vi "Show Block Diagram.vi"(8 "error in":errorcluster, 11 "VI in":refnum<vi>) -> (0 "error out":errorcluster)   [LabVIEW 2014, in "Chart Module.lvlib"]
uses:
  Chart Module.lvlib
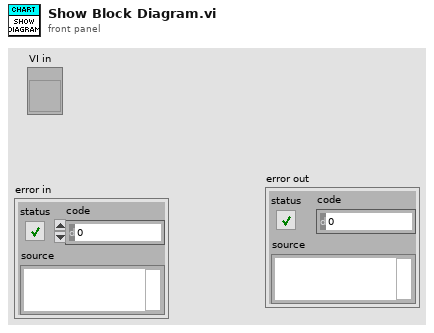
[diagram p1: front panel]
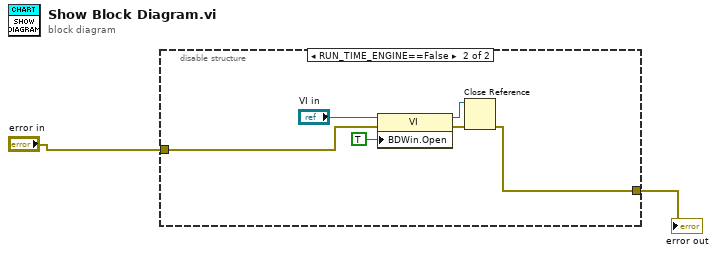
[diagram p0: block diagram]
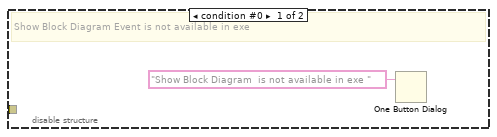
[diagram p2: hidden frame]
diagram:
  n1 = disable-structure shown="RUN_TIME_ENGINE==False" {
    disable-tunnel: [_ w5] -> w2
    disable-tunnel: "error in" -> [_ w4]
    frame condition #0 {
      # "Show Block Diagram Event is not available in exe"
      n2 = One Button Dialog(message="Show Block Diagram  is not available in exe ") -> ()  [unwired: 1 in, 1 out]
    }
    frame condition #1 (active) {
      n3 = property class="VI"(reference="VI in", error in=w4, "BDWin.Open"=TRUE ("Block Diagram Window:Open")) -> (reference out=w7:refnum<vi>, error out=w6:errorcluster)
      n4 = Close Reference(reference=w7, error in (no error)=w6) -> (error out=w5:errorcluster)
    }
  }
  "error out" <- w2
